vi "testLua_xmove.vi"() -> ()   [LabVIEW 2011]
panel:
  out "lua_Number":dbl
  out "lua_type":i32(ring) items=["LUA_TNONE"=-1, "LUA_TNIL"=0, "LUA_TBOOLEAN"=1, "LUA_TLIGHTUSERDATA"=2, "LUA_TNUMBER "=3, "LUA_TSTRING"=4, "LUA_TTABLE"=5, "LUA_TFUNCTION"=6, "LUA_TUSERDATA"=7, "LUA_TTHREAD"=8, "LUA_NUMTAGS "=9]
  in  "get":bool
  in  "const char *name":string
  in  "lua_State *from":u64
  in  "停止":bool
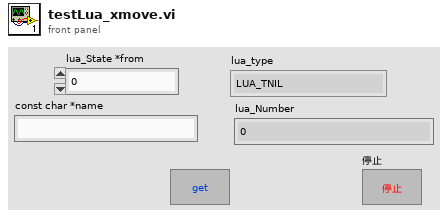
[diagram p1: front panel]
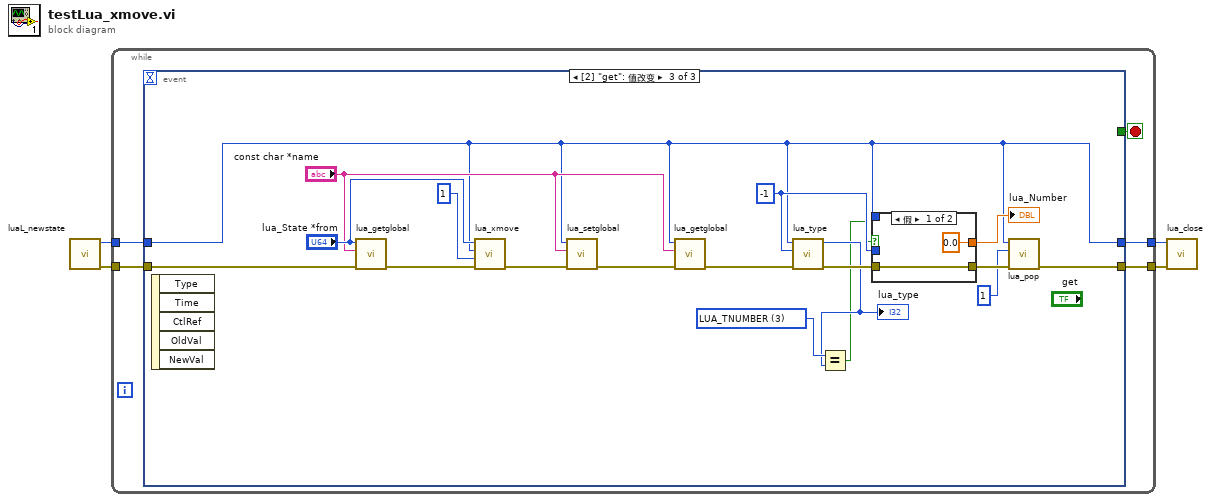
[diagram p0: block diagram]
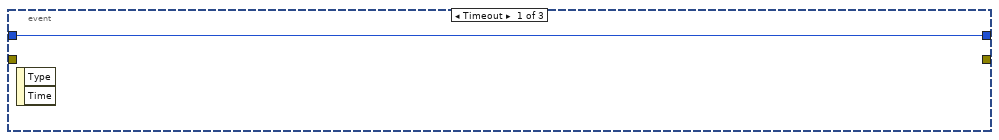
[diagram p2: hidden frame]
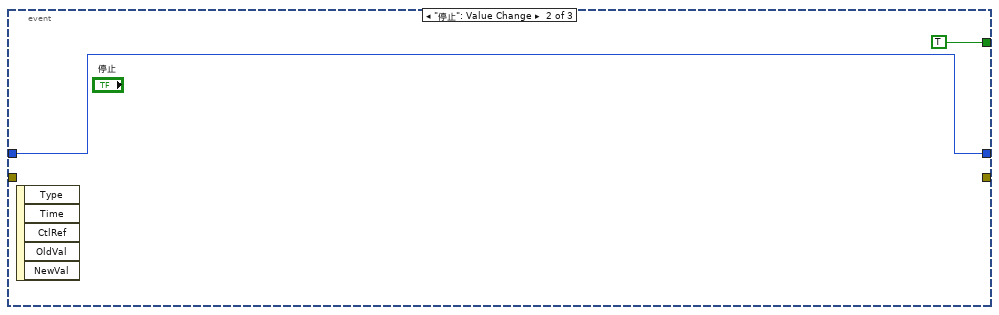
[diagram p3: hidden frame]
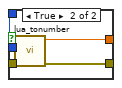
[diagram p4: hidden frame]
diagram:
  n1 = call "luaL_newstate.vi"() -> ("error out"=w3:errorcluster, "lua_State *luaL_newstate"=w4:u64)  [unwired: 10 in]
  n2 = while {
    tunnel: w4 -> [w7]
    tunnel: w3 -> [w8]
    tunnel: [w6] -> w2
    tunnel: [w5] -> w1
    stop <- w9 stop-if-true
    n3 = event shown="[2] \"get\": 值改变" {
      selector: _ -> [_ _ _]
      dyn-events: _ -> [_ _ _]
      timeout: _ -> [_ _ _]
      tunnel: [_ TRUE _] -> w9
      tunnel: w8 -> [_ _ w30]
      tunnel: w7 -> [w10 w11 w16]
      tunnel: [_ _ w17] -> w6
      tunnel: [w10 w11 w16] -> w5
      event Timeout {
        n4 = event-data() -> ()  [unwired: 1 in, 2 out]
      }
      event "停止": Value Change {
        n5 = event-data() -> ()  [unwired: 1 in, 5 out]
      }
      event "get": Value Change {
        w15 = 3 items=["LUA_TNONE"=-1, "LUA_TNIL"=0, "LUA_TBOOLEAN"=1, "LUA_TLIGHTUSERDATA"=2, "LUA_TNUMBER "=3, "LUA_TSTRING"=4, "LUA_TTABLE"=5, "LUA_TFUNCTION"=6, "LUA_TUSERDATA"=7, "LUA_TTHREAD"=8, "LUA_NUMTAGS "=9] ("lua_type")
        w21 = -1 ("int index")
        n6 = event-data() -> ()  [unwired: 1 in, 5 out]
        n7 = call "lua_getglobal.vi"("error in"=w30, "const char *name"="const char *name", "lua_State *L"="lua_State *from") -> ("error out"=w29:errorcluster)  [unwired: 8 in]
        n8 = call "lua_xmove.vi"("error in"=w29, "int n"=1, "lua_State *to"=w16, "lua_State *from"="lua_State *from") -> ("error out"=w26:errorcluster)  [unwired: 7 in]
        n9 = call "lua_setglobal.vi"("error in"=w26, "s"="const char *name", "lua_State *L"=w16) -> ("error out"=w25:errorcluster)  [unwired: 8 in]
        n10 = call "lua_getglobal.vi"("error in"=w25, "const char *name"="const char *name", "lua_State *L"=w16) -> ("error out"=w23:errorcluster)  [unwired: 8 in]
        n11 = call "lua_type.vi"("error in"=w23, "int index"=w21, "lua_State *L"=w16) -> ("error out"=w22:errorcluster, "lua_type"=w14:i32)  [unwired: 7 in]
        "lua_type" <- w14
        n12 = Equal?(x=w15, y=w14) -> (x = y?=w13:bool)
        n13 = case shown="假" w13 {
          tunnel: w22 -> [w31 w37]
          tunnel: w21 -> [_ w36]
          tunnel: [w31 w35] -> w20
          tunnel: [0.0 ("lua_Number") w34] -> w19
          tunnel: w16 -> [_ w33]
          frame False {
          }
          frame True {
            n14 = call "lua_tonumber.vi"("error in"=w37, "index"=w36, "lua_State *L"=w33) -> ("error out"=w35:errorcluster, "lua_Number"=w34:dbl)  [unwired: 7 in]
          }
        }
        "lua_Number" <- w19
        n15 = call "lua_pop.vi"("error in"=w20, "n"=1, "lua_State *L"=w16) -> ("error out"=w17:errorcluster)  [unwired: 8 in]
      }
    }
  }
  n16 = call "lua_close.vi"("error in"=w2, "lua_State *L"=w1) -> ()  [unwired: 9 in, 1 out]
